vi "Test-Meas HV Sweep.vi"(5 "Delay before 1st measurment":dbl=0.003 format="%#_13p", 7 "script name":string="HVSweep", 8 "error in (no error)":errorcluster, 9 "Publishable IDs":string[](array[string])=["PostFuse_HV29", "PostFuse_HV30", "PostFuse_HV31"], 10 "Pins":string[](array[string])=["HV"], 11 "Semiconductor Module Context":T1) -> (0 "error out":errorcluster)   [LabVIEW 2013]
uses:
  <vilib>/NI_TestStand_SemiconductorModule/NI_TestStand_Semiconductor_Module.lvlibp/PinMap/General/SemiconductorModuleContext.ctl
  <instrlib>/niHSDIO/niHSDIO.llb/niHSDIO_ctl Trigger Script - trigID Values (Ring).ctl
  <instrlib>/niDCPower/nidcpower.llb/niDCPower Measurement Type.ctl
  <vilib>/NI_TestStand_SemiconductorModule/NI_TestStand_Semiconductor_Module.lvlibp/PinMap/DC Power/PinsToNIDCPowerSessions.vi
  <vilib>/NI_TestStand_SemiconductorModule/NI_TestStand_Semiconductor_Module.lvlibp/PinMap/General/Publish/PublishDataDouble2D.vi
  <vilib>/NI_TestStand_SemiconductorModule/NI_TestStand_Semiconductor_Module.lvlibp
panel:
  out "Measurements":dbl[][](array[numeric])
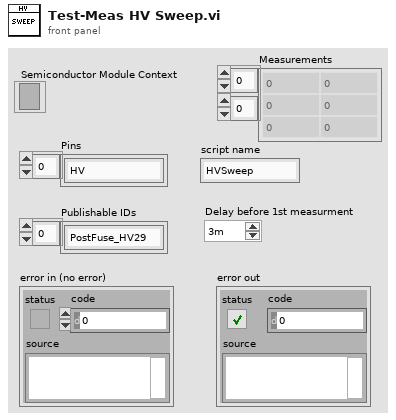
[diagram p1: front panel]
types:
  T1 = typedef "NI_TestStand_Semiconductor_Module.lvlibp/SemiconductorModuleContext.ctl" = refnum<k7>
  T2 = typedef "niHSDIO_ctl Trigger Script - trigID Values (Ring).ctl" = string
  T3 = typedef "niDCPower Measurement Type.ctl" = i32
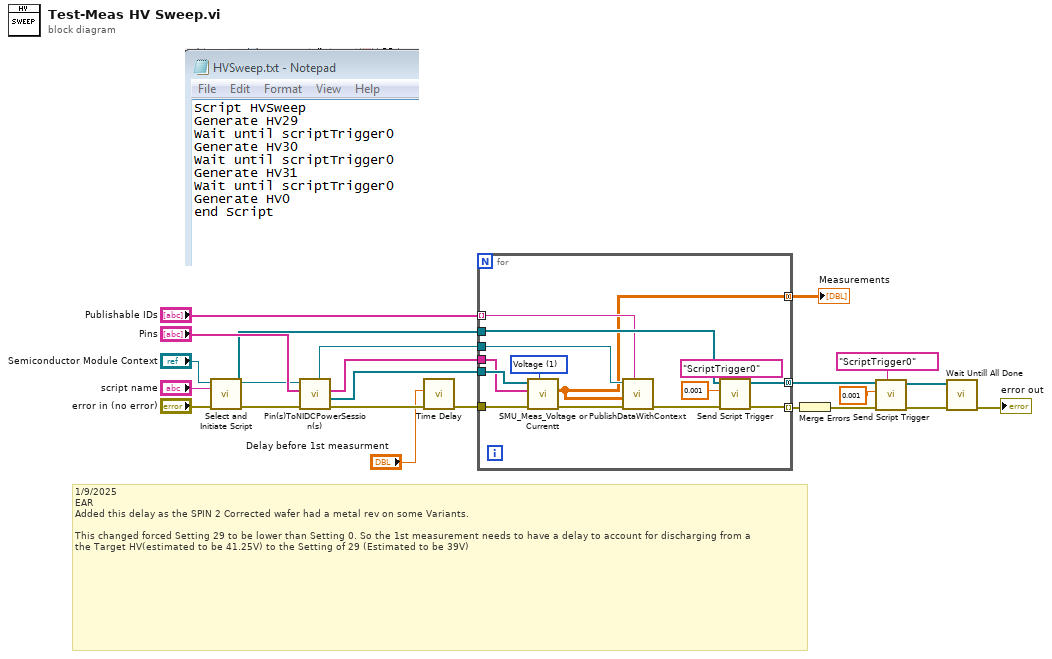
[diagram p0: block diagram]
diagram:
  # "1/9/2025\nEAR\nAdded this delay as the SPIN 2 Corrected wafer had a metal rev on some Variants.\n\nThis changed forced Setting 29 to be lower than Setting 0. So the 1st measurement needs to have a delay to account for discharging from a\nthe Target HV(estimated to be 41.25V) to the Setting of 29 (Estimated to be 39V)"
  n1 = call "Select and Initiate Script.vi"("error in (no error)"="error in (no error)", "script name"="script name", "Semiconductor Module Context"="Semiconductor Module Context") -> ("error out"=w16:errorcluster, "HSDIO GEN Sessions Out"=w12:refnum<k15>[], "Semiconductor Module Context Out"=w14:T1)  [unwired: 6 in]
  n2 = call-poly <vilib>:"Pin(s)ToNIDCPowerSession(s).vi"("error in (no error)"=w16, "Pins"="Pins", "Semiconductor Module Context"=w14) -> ("error out"=w2:errorcluster, "Instrument Sessions"=w22:refnum<k15>[], "Channel Lists"=w20:string[], "Pin Query Context"=w21:refnum<class "MultiplePinMultipleSessionQueryContext.lvclass">)  [unwired: 4 in, 1 out]
  n3 = call "Time Delay"("error in (no error)"=w2, "Delay Time (s)"="Delay before 1st measurment") -> ("error out"=w3:errorcluster)  [unwired: 9 in]
  n4 = for {
    tunnel: w3 -> [w37]
    tunnel: w22 -> [w36]
    tunnel: w21 -> [w34]
    tunnel: [w29] -> w11 mode=indexing
    tunnel: w20 -> [w33]
    tunnel: "Publishable IDs" -> [w26] mode=indexing
    tunnel: w12 -> [w27]
    tunnel: [w25] -> w7 mode=concatenating
    tunnel: [w24] -> w4 mode=concatenating
    w32 = T3 1 items=["Current", "Voltage"] ("measurement type")
    n5 = call "SMU_Meas_Voltage or Currentt.vi"("measurement type"=w32, "error in (no error)"=w37, "Channel Lists"=w33, "DCPower Sessions In"=w36) -> ("error out"=w35:errorcluster, "Measurement"=w24:dbl[][])  [unwired: 5 in, 1 out]
    n6 = call-poly <vilib>:"PublishDataWithContext.vi"("Published Data Id"=w26, "error in (no error)"=w35, "Data In"=w24, "Pin Query Context"=w34) -> ("error out"=w30:errorcluster)  [unwired: 6 in, 1 out]
    n7 = call "Send Script Trigger.vi"("trigger id (script trigger 0)"=T2 "ScriptTrigger0", "error in (no error)"=w30, "Delay Time (s)"=0.001, "HSDIO Sessions In"=w27) -> ("error out"=w29:errorcluster, "HSDIO Sessions Out"=w25:refnum<k15>[])  [unwired: 6 in]
  }
  "Measurements" <- w4
  n8 = Merge Errors(w11) -> (w10:errorcluster)
  n9 = call "Send Script Trigger.vi"("trigger id (script trigger 0)"=T2 "ScriptTrigger0", "error in (no error)"=w10, "Delay Time (s)"=0.001, "HSDIO Sessions In"=w7) -> ("error out"=w9:errorcluster, "HSDIO Sessions Out"=w6:refnum<k15>[])  [unwired: 6 in]
  n10 = call "Wait Untill All Done.vi"("error in (no error)"=w9, "HSDIO Sessions In"=w6) -> ("error out"=→"error out":errorcluster)  [unwired: 8 in, 1 out]
